vi "Generate Descriptor VI.vi"(8 "error in (no error)":errorcluster, 10 "Descriptor Strings":string[](array[string]), 11 "Library":refnum<vi>) -> (0 "error out":errorcluster, 3 "Library":refnum<vi>)   [LabVIEW 2019, in "gRPC Template Creation Utility.lvlib"]
uses:
  gRPC Template Creation Utility.lvlib
  <vilib>/gRPC/gRPC Server and Client Template [2]/gRPC Scripting Tools/gRPC Template Creation Utility-release.lvlib
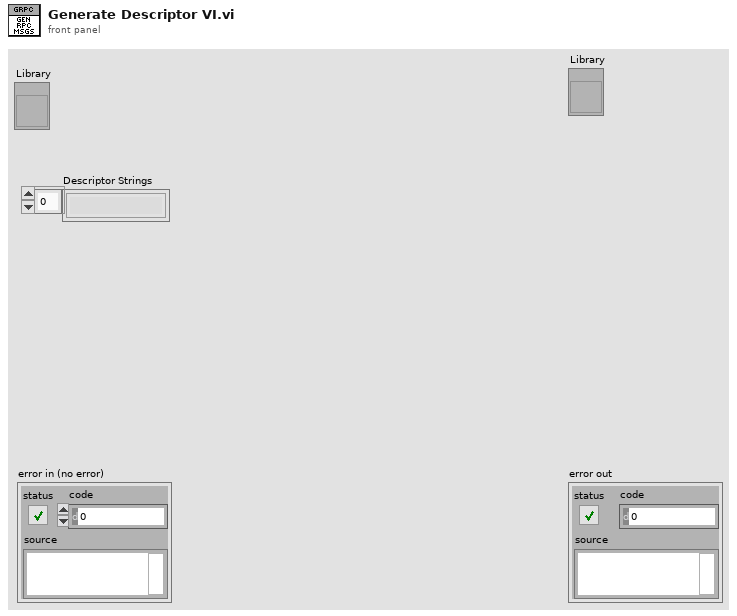
[diagram p1: front panel]
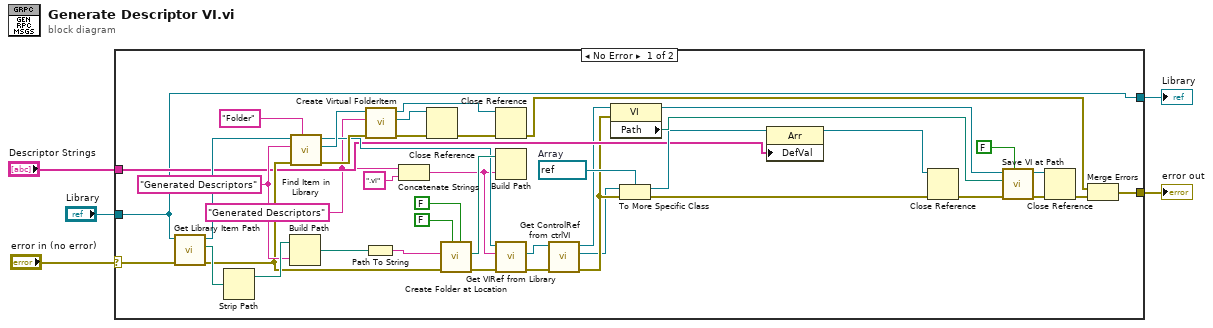
[diagram p0: block diagram]
diagram:
  n1 = case shown="No Error" "error in (no error)" {
    selector: "error in (no error)" -> [w17 w50]
    tunnel: [w16 w50] -> w5
    tunnel: [w13 w49] -> w4
    tunnel: "Library" -> [w13 w49]
    tunnel: "Descriptor Strings" -> [w15 _]
    frame No Error {
      w12 = refnum<vi> refnum  # Array
      w14 = "Generated Descriptors" ("Folder Name")
      w36 = "Generated Descriptors" ("Item Name")
      n2 = call <vilib>:"Get Library Item Path.vi"("error in (no error)"=w17, "Library"=w13) -> ("error out"=w35:errorcluster, "Path"=w43:path, "Library"=w37:refnum<vi>)  [unwired: 7 in]
      n3 = Strip Path(path=w43) -> (stripped path=w44:path)  [unwired: 1 out]
      n4 = Build Path(base path=w44, name or relative path=w36) -> (appended path=w18:path)
      n5 = call <vilib>:"Find Item in Library.vi"("Item Type"="Folder", "error in (no error)"=w35, "Item Name"=w36, "Library item in"=w37) -> ("error out"=w34:errorcluster, "Project Item (Library Item)"=w38:refnum<vi>, "Library item out"=w29:refnum<vi>)  [unwired: 4 in, 1 out]
      n6 = Path To String(path=w18) -> (string=w47:string)
      n7 = call <vilib>:"Create Virtual FolderItem.vi"("error in (no error)"=w34, "Folder Name"=w14, "ProjectItem in"=w38) -> ("error out"=w25:errorcluster, "FolderItem reference out"=w26:refnum<vi>, "ProjectItem out"=w28:refnum<vi>)  [unwired: 5 in, 1 out]
      n8 = Concatenate Strings(w14, ".vi" ("string")) -> (w23:string)
      n9 = Close Reference(reference=w26, error in (no error)=w25) -> (error out=w32:errorcluster)
      n10 = call <vilib>:"Create Folder at Location.vi"("Override existing (F)"=FALSE, "Use Relative (F)"=FALSE ("Use Relative"), "Error In"=w35, "Path"=w47) -> ("Error Out"=w46:errorcluster, "Full path out"=w48:path)  [unwired: 5 in, 1 out]
      n11 = Close Reference(reference=w28, error in (no error)=w32) -> (error out=w31:errorcluster)
      n12 = Build Path(base path=w48, name or relative path=w23) -> ()  [unwired: 1 out]
      n13 = call <vilib>:"Get VIRef from Library.vi"("error in (no error)"=w46, "Item Name"=w23, "Library"=w29) -> ("error out"=w10:errorcluster, "VIref out"=w11:refnum<vi>)  [unwired: 5 in, 2 out]
      n14 = call <vilib>:"Get ControlRef from ctrlVI.vi"("error in (no error)"=w10, "VI ref in"=w11) -> ("error out"=w8:errorcluster, "Control ref out"=w7:refnum<vi>, "VI ref out"=w9:refnum<vi>)  [unwired: 7 in]
      n15 = property class="VI"(reference=w9, error in=w8) -> (reference out=w6:refnum<vi>, "Path"=w27:path)  [unwired: 1 out]
      n16 = To More Specific Class(target class=w12, reference=w7, error in=w8) -> (specific class reference=w22:refnum<vi>, error out=w21:errorcluster)
      n17 = property class="Arr"(reference=w22, "DefVal"=w15) -> (reference out=w20:refnum<vi>)  [unwired: 1 in, 1 out]
      n18 = Close Reference(reference=w20, error in (no error)=w21) -> (error out=w30:errorcluster)
      n19 = call <vilib>:"Save VI at Path.vi"("Override Existing? (T)"=FALSE, "error in (no error)"=w30, "Path"=w27, "VI in"=w6) -> ("error out"=w41:errorcluster, "VI out"=w40:refnum<vi>)  [unwired: 5 in, 1 out]
      n20 = Close Reference(reference=w40, error in (no error)=w41) -> (error out=w33:errorcluster)
      n21 = Merge Errors(w31, w33) -> (w16:errorcluster)
    }
    frame Error {
    }
  }
  "error out" <- w5
  "Library" <- w4
